vi "Get Voices.vi"(4 "error out":errorcluster, 5 "OptionalAttributes":string, 6 "RequiredAttributes":string, 7 "SpeechLib.ISpeechVoice (In)":refnum<k7>) -> (0 "error in (no error)":errorcluster, 1 "Voice Names":string[](array[string]), 2 "GetVoices":refnum<k7>, 3 "SpeechLib.ISpeechVoice (Out)":refnum<k7>)   [LabVIEW 2018]
doc: "This SubVI calls the Microsoft Speech SDK 5.1 software and loads the voices available into an output array for use by the LVTTS.vi"
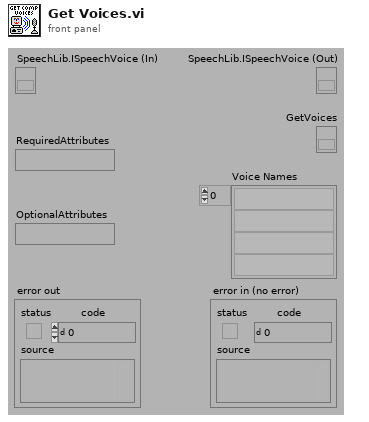
[diagram p1: front panel]
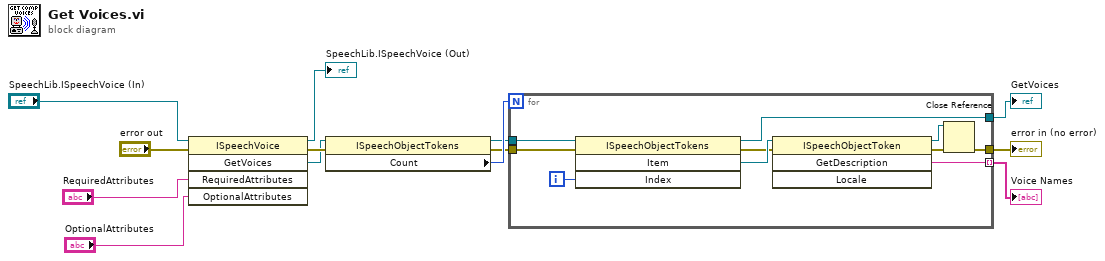
[diagram p0: block diagram]
diagram:
  n1 = invoke class="ISpeechVoice" method="GetVoices"(reference="SpeechLib.ISpeechVoice (In)", error in="error out", "RequiredAttributes"="RequiredAttributes", "OptionalAttributes"="OptionalAttributes") -> (reference out=→"SpeechLib.ISpeechVoice (Out)":refnum<k7>, error out=w7:errorcluster, "GetVoices"=w6:refnum<k7>)  [unwired: 1 in, 2 out]
  n2 = property class="ISpeechObjectTokens"(reference=w6, error in=w7) -> (reference out=w9:refnum<k7>, error out=w8:errorcluster, "Count"=w11:i32)
  n3 = for {
    N: w11 -> [_]
    tunnel: [w14] -> w5
    tunnel: w8 -> [w20]
    tunnel: w9 -> [w19]
    tunnel: [w18] -> w10
    tunnel: [w17] -> w12 mode=indexing
    i -> [w22]
    n4 = invoke class="ISpeechObjectTokens" method="Item"(reference=w19, error in=w20, "Index"=w22) -> (reference out=w18:refnum<k7>, error out=w16:errorcluster, "Item"=w23:refnum<k7>)  [unwired: 1 in, 1 out]
    n5 = invoke class="ISpeechObjectToken" method="GetDescription"(reference=w23, error in=w16) -> (reference out=w21:refnum<k7>, error out=w15:errorcluster, "GetDescription"=w17:string)  [unwired: 2 in, 1 out]
    n6 = Close Reference(reference=w21, error in (no error)=w15) -> (error out=w14:errorcluster)
  }
  "Voice Names" <- w12
  "GetVoices" <- w10
  "error in (no error)" <- w5
